vi "cst--X_axis_units.vi"() -> ()   [LabVIEW 2013]
panel:
  in  "X Axis Unit (ref)":string[](array[string])
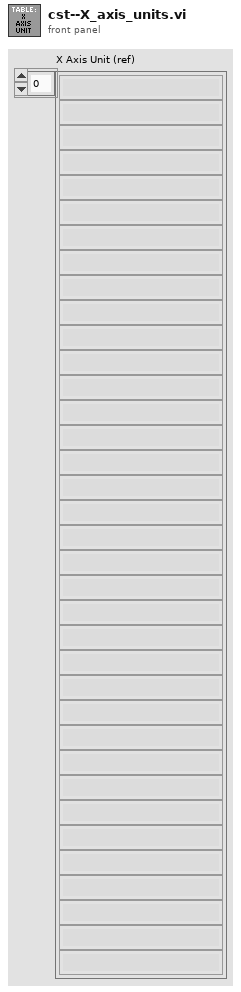
[diagram p1: front panel]
diagram:
